vi "DFD FXP MRate Postprocessing (I32, nCh).vi"(5 "input range":dbl=1.0, 6 "history in":i32[](array[numeric]), 7 "# channels":i32=1, 8 "error in (no error)":errorcluster, 10 "multirate filter":T1={"mMRate_Structure"=enum."IIR", "mMRate_Mode"=0, "mMRate_Factor"=-1, "mMRate_FIRParams"={"mMRate_FIR_H"=[], "mMRate_FIR_IsNyquist?"=FALSE, "mMRate_FIR_IsSymmetric?"=FALSE}, "mMRate_CICParams"={"mMRate_CIC_#Stage"=0, "mMRate_CIC_Lag"=0, "mMRate_CIC_Type"=enum."Lowpass"}, "mMRate_Order"=0, "mMRate_Version"="2.0", "mMRate_Comments"="", "mMRate_RationalFactor"={"mMRate_L"=-1, "mMRate_M"=-1}, "mMRate_Fs"=1.0, "mMRate_Quantized?"=FALSE, "mMRate_QFilterGain"=1.0, "mMRate_CoefWl"=16, "mMRate_Scaling"={"mMRate_ScaleByPowerOf2?"=FALSE, "mMRate_ScaleType"=enum."No Norm"}, "mMRate_InputWl"=16, "mMRate_OutputWl"=16, "mMRate_OutputMode"=enum."Truncation", "mMRate_MultMode"=enum."Truncated", "mMRate_BitPruning"=FALSE, "mMRate_GainWl"=16, "mMRate_OutputFwl"=0, "mMRate_SumIwl"=0, "mMRate_InputIwl "=16, "mMRate_SumWl"=32, "mMRate_CoefIwl"=0} {"mMRate_SumWl" min=1 max=32 step=1; "mMRate_InputIwl" min=1 max=32 step=1; "mMRate_GainWl" min=1 max=32 step=1; "mMRate_OutputWl" min=1 max=32 step=1; "mMRate_InputWl" min=1 max=32 step=1; "mMRate_CoefWl" min=1 max=32 step=1; "mMRate_Mode" items=["Default"=-1, "No Rate Change"=0, "Interpolation"=1, "Decimation"=2, "Interpolated"=3, "Rational"=4]}, 11 "signal in":i32[](array[numeric]) format="%.0x") -> (0 "error out":errorcluster, 3 "signal out":dbl[][](array[numeric]), 4 "history out":i32[](array[numeric]))   [LabVIEW 2017, in "NI_DigFilterLicensed.lvlib"]
doc: "Converts the output signal of a fixed-point multirate filter from an integer, fixed-point representation to a floating-point representation. You must manually select the polymorphic instance you want to use."
uses:
  <vilib>/addons/Digital Filter Design/NI_DigFilterLicensed.lvlib
  <vilib>/addons/Digital Filter Design/_Objects.llb/DFD Multirate Filter Obj.ctl
  <vilib>/addons/Digital Filter Design/_Objects.llb/DFD Multirate Mode.ctl
  <vilib>/addons/Digital Filter Design/_Objects.llb/DFD Coef Norm Type.ctl
  <vilib>/addons/Digital Filter Design/_Objects.llb/DFD Round-off Mode.ctl
  <vilib>/addons/Digital Filter Design/_Objects.llb/DFD FXP MRate Multiply Mode.ctl
  <vilib>/addons/Digital Filter Design/_Misc.llb/dfd_Error Handlers (Single).vi
  <vilib>/addons/Digital Filter Design/NI_DigFilter_FXP.lvlib
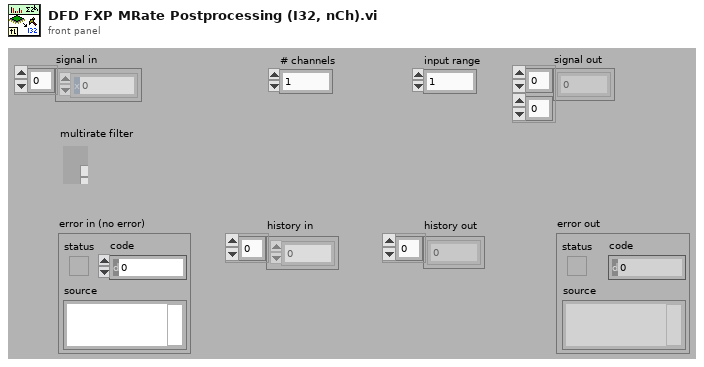
[diagram p1: front panel]
types:
  T1 = typedef "NI_DigFilterLicensed.lvlib/DFD Multirate Filter Obj.ctl" = cluster{"mMRate_Structure":enum16{"CIC", "FIR", "IIR", "Lattice"}, "mMRate_Mode":T2, "mMRate_Factor":i32, "mMRate_FIRParams":cluster{"mMRate_FIR_H":dbl[], "mMRate_FIR_IsNyquist?":bool, "mMRate_FIR_IsSymmetric?":bool}, "mMRate_CICParams":cluster{"mMRate_CIC_#Stage":i32, "mMRate_CIC_Lag":i32, "mMRate_CIC_Type":enum16{"Lowpass", "Highpass"}}, "mMRate_Order":i32, "mMRate_Version":string, "mMRate_Comments":string, "mMRate_RationalFactor":cluster{"mMRate_L":i32, "mMRate_M":i32}, "mMRate_Fs":dbl, "mMRate_Quantized?":bool, "mMRate_QFilterGain":dbl, "mMRate_CoefWl":i16, "mMRate_Scaling":cluster{"mMRate_ScaleByPowerOf2?":bool, "mMRate_ScaleType":T3}, "mMRate_InputWl":i16, "mMRate_OutputWl":i16, "mMRate_OutputMode":T4, "mMRate_MultMode":T5, "mMRate_BitPruning":bool, "mMRate_GainWl":i16, "mMRate_OutputFwl":i16, "mMRate_SumIwl":i16, "mMRate_InputIwl ":i16, "mMRate_SumWl":i16, "mMRate_CoefIwl":i16}
  T2 = typedef "NI_DigFilterLicensed.lvlib/DFD Multirate Mode.ctl" = i16
  T3 = typedef "NI_DigFilterLicensed.lvlib/DFD Coef Norm Type.ctl" = enum16{"No Norm", "Time Domain 1-Norm", "Time Domain 2-Norm", "Time Domain Inf-Norm"}
  T4 = typedef "NI_DigFilterLicensed.lvlib/DFD Round-off Mode.ctl" = enum16{"Nearest", "Truncation"}
  T5 = typedef "NI_DigFilterLicensed.lvlib/DFD FXP MRate Multiply Mode.ctl" = enum16{"Truncated", "Full"}
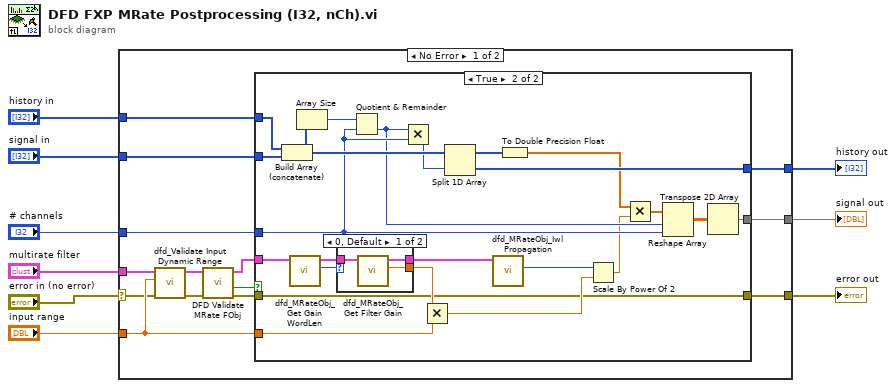
[diagram p0: block diagram]
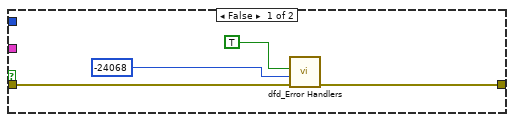
[diagram p2: hidden frame]
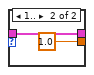
[diagram p3: hidden frame]
diagram:
  n1 = case shown="No Error" "error in (no error)" {
    selector: "error in (no error)" -> [w10 w55]
    tunnel: "signal in" -> [w22 _]
    tunnel: "history in" -> [w21 _]
    tunnel: [w20 _] -> w7
    tunnel: [w19 _] -> w6
    tunnel: "# channels" -> [w18 _]
    tunnel: "multirate filter" -> [w17 _]
    tunnel: [w15 w55] -> w3
    tunnel: "input range" -> [w12 _]
    frame No Error {
      n2 = call <vilib>:"dfd_Validate Input Dynamic Range.vi"("error in (no error)"=w10, "input range"=w12) -> ("error out"=w13:errorcluster)  [unwired: 9 out]
      n3 = call <vilib>:"DFD Validate MRate FObj.vi"("error in (no error)"=w13, "multirate filter in"=w17) -> ("error out"=w11:errorcluster, "is valid FXP?"=w14:bool, "multirate filter out"=w16:T1)  [unwired: 7 out]
      n4 = case shown="True" w14 {
        tunnel: w22 -> [_ w48]
        tunnel: w21 -> [_ w47]
        tunnel: [_ w44] -> w20
        tunnel: [_ w41] -> w19
        tunnel: w18 -> [_ w40]
        tunnel: w16 -> [_ w30]
        tunnel: w12 -> [_ w33]
        tunnel: w11 -> [w24 w32]
        tunnel: [w23 w32] -> w15
        frame False {
          n5 = call-poly <vilib>:"dfd_Error Handlers.vi"("error in (no error)"=w24, "error code"=-24068 ("ERR_INVALID_FXP_MRATE"), "condition failed?"=TRUE) -> ("error out"=w23:errorcluster)  [unwired: 8 out]
        }
        frame True {
          n6 = Build Array (concatenate)(w47, w48) -> (w46:i32[])
          n7 = call <vilib>:"dfd_MRateObj_Get Gain WordLen.vi"("multirate filter in"=w30) -> ("gain wl"=w28:i16, "dup multirate filter"=w29:T1)  [unwired: 9 out]
          n8 = Array Size(array=w46) -> (size(s)=w49:i32)
          n9 = case shown="0, Default" w28 {
            tunnel: [w52 1.0 ("gain")] -> w34
            tunnel: [w51 w54] -> w31
            tunnel: w29 -> [w50 w54]
            frame 0, Default {
              n10 = call <vilib>:"dfd_MRateObj_Get Filter Gain.vi"("multirate filter in"=w50) -> ("gain"=w52:dbl, "dup multirate filter"=w51:T1)  [unwired: 9 out]
            }
            frame 1.. {
            }
          }
          n11 = Quotient & Remainder(x=w49, y=w40) -> (floor(x/y)=w39:i32)  [unwired: 1 out]
          n12 = Multiply(x=w39, y=w40) -> (x*y=w45:i32)
          n13 = Multiply(x=w34, y=w33) -> (x*y=w37:dbl)
          n14 = Split 1D Array(array=w46, index=w45) -> (first subarray=w38:i32[], second subarray=w44:i32[])
          n15 = call <vilib>:"dfd_MRateObj_Iwl Propagation.vi"("multirate filter"=w31) -> ("Actual Output -fwl"=w27:i16)  [unwired: 10 out]
          n16 = To Double Precision Float(number=w38) -> (double precision float=w36:dbl[])
          n17 = Scale By Power Of 2(n=w27, x=w37) -> (x*2^n=w35:dbl)
          n18 = Multiply(x=w36, y=w35) -> (x*y=w43:dbl[])
          n19 = Reshape Array(w43, w39, w40) -> (w42:dbl[][])
          n20 = Transpose 2D Array(2D array=w42) -> (transposed array=w41:dbl[][])
        }
      }
    }
    frame Error {
    }
  }
  "signal out" <- w6
  "error out" <- w3
  "history out" <- w7
